vi "Worksheet to Dictionaries.vi"(8 "error in (no error)":errorcluster, 11 "Worksheet Data":T1) -> (0 "error out":errorcluster, 3 "Dictionaries Out":refnum<class "String Database.lvclass">[](array[class]))   [LabVIEW 2016, in "QPA TCF Parser.lvlib" / "QPA TCF Parser.lvclass"]
uses:
  QPA TCF Parser.lvclass
  Controls/Worksheet Data.ctl
  Plugins/String Database.lvlibp/String Database.lvclass
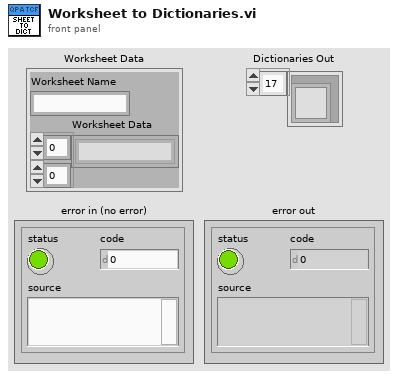
[diagram p1: front panel]
types:
  T1 = typedef "QPA TCF Parser.lvlib/QPA TCF Parser.lvclass/Worksheet Data.ctl" = cluster{"Worksheet Name":string, "Worksheet Data":string[][]}
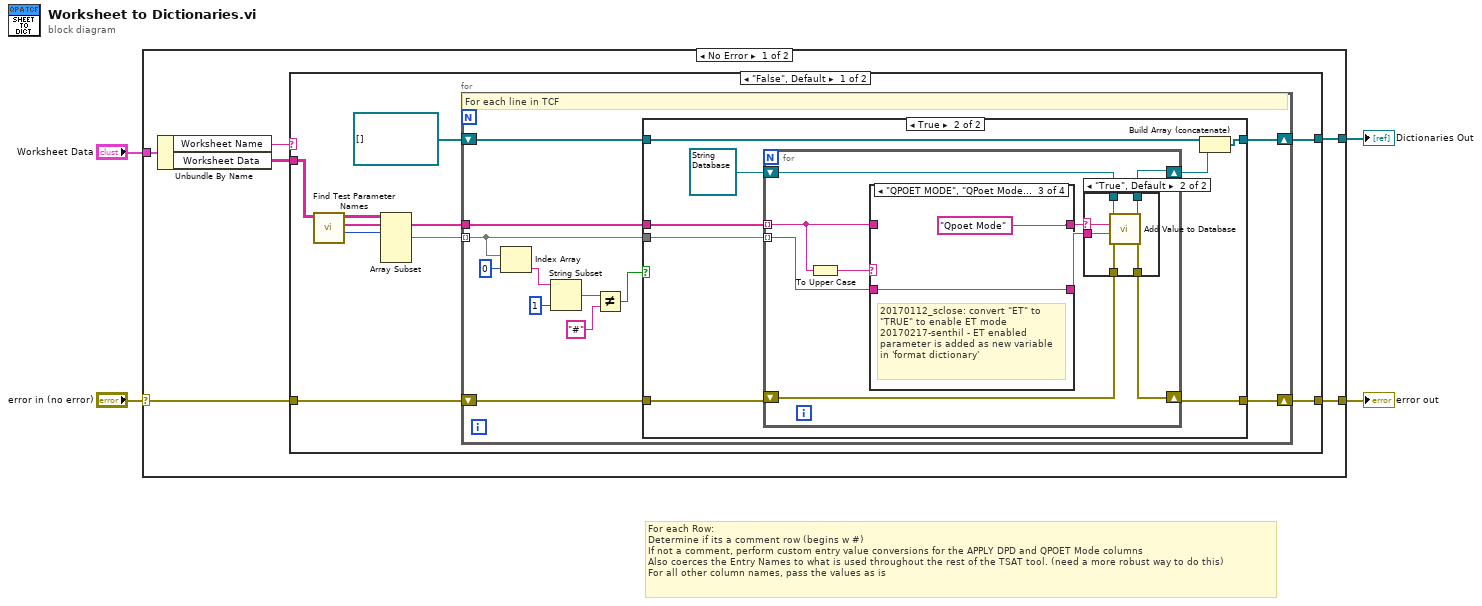
[diagram p0: block diagram]
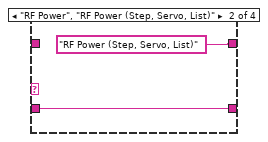
[diagram p4: hidden frame]
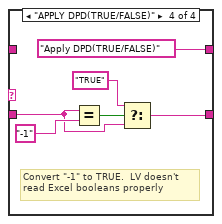
[diagram p5: hidden frame]
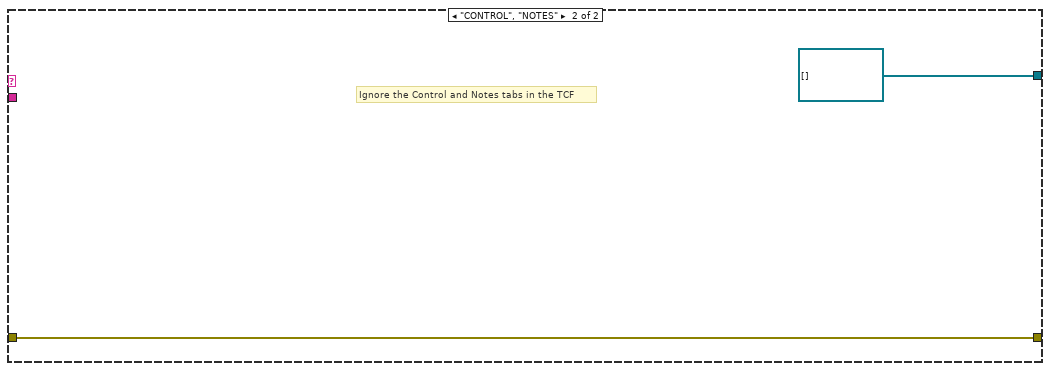
[diagram p7: hidden frame]
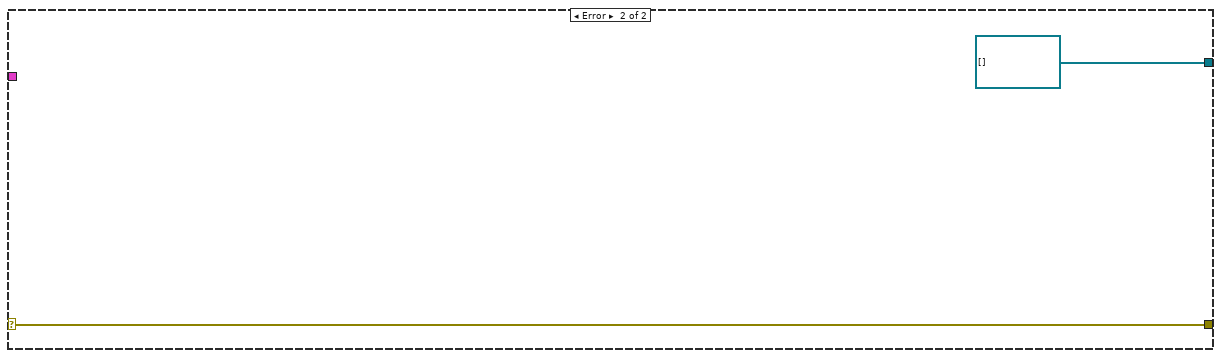
[diagram p8: hidden frame]
diagram:
  # "For each Row:\nDetermine if its a comment row (begins w #)\nIf not a comment, perform custom entry value conversions for the APPLY DPD and QPOET Mode columns\nAlso coerces the Entry Names to what is used throughout the rest of the TSAT tool. (need a more robust way to do this)\nFor all other column names, pass the values as is"
  n1 = case shown="No Error" "error in (no error)" {
    selector: "error in (no error)" -> [w9 w73]
    tunnel: [w10 w73] -> w4
    tunnel: "Worksheet Data" -> [w6 _]
    tunnel: [w5 refnum<class "String Database.lvclass">[] [] ("Dictionaries Out")] -> w1
    frame No Error {
      n2 = Unbundle By Name(w6) -> ("Worksheet Name"=w7:string, "Worksheet Data"=w8:string[][])
      n3 = case shown="\"False\", Default" w7 {
        tunnel: w8 -> [w19 _]
        tunnel: w9 -> [w14 w71]
        tunnel: [w13 w71] -> w10
        tunnel: [w11 refnum<class "String Database.lvclass">[] [] ("Dictionaries Out")] -> w5
        frame "False", Default {
          n4 = call "Find Test Parameter Names.vi"("Worksheet Data"=w19) -> ("Test Parameter Row Index"=w17:i32, "Test Parameters"=w15:string[], "Worksheet Data Out"=w18:string[][])  [unwired: 8 in]
          n5 = Array Subset(array=w18, index (row)=w17) -> (w16:string[][])  [unwired: 3 in]
          n6 = for {
            tunnel: w16 -> [w28] mode=indexing
            tunnel: w15 -> [w31]
            shift-right: [w29] -> w13
            shift-left: w14 -> [w30]
            shift-right: [w20] -> w11
            shift-left: refnum<class "String Database.lvclass">[] [] -> [w21]
            # "For each line in TCF"
            n7 = Index Array(array=w28, index=0) -> (element=w26:string)
            n8 = String Subset(string=w26, length (rest)=1 ("length (rest)")) -> (substring=w24:string)  [unwired: 1 in]
            n9 = Not Equal?(x=w24, y="#") -> (x != y?=w22:bool)
            n10 = case shown="True" w22 {
              tunnel: w31 -> [_ w41]
              tunnel: w30 -> [w33 w38]
              tunnel: [w33 w40] -> w29
              tunnel: w28 -> [_ w39]
              tunnel: w21 -> [w32 w35]
              tunnel: [w32 w34] -> w20
              frame False {
                # "Do Nothing on # comment"
              }
              frame True {
                n11 = for {
                  tunnel: w41 -> [w43] mode=indexing
                  tunnel: w39 -> [w46] mode=indexing
                  shift-right: [w48] -> w40
                  shift-left: w38 -> [w49]
                  shift-right: [w47] -> w36
                  shift-left: refnum<class "String Database.lvclass"> refnum ("String Database out") -> [w50]
                  n12 = To Upper Case(1:w43) -> (0:w44:string)
                  n13 = case shown="\"QPOET MODE\", \"QPoet Mode (Bypass, APT, EPT, ET)\"" w44 {
                    tunnel: w46 -> [w52 w54 w55 w59]
                    tunnel: [w52 w54 w55 w60] -> w45
                    tunnel: w43 -> [w51 _ _ _]
                    tunnel: [w51 "RF Power (Step, Servo, List)" ("Entry Name") "Qpoet Mode" ("Entry Name") "Apply DPD(TRUE/FALSE)" ("Entry Name")] -> w42
                    frame "", Default {
                    }
                    frame "RF Power", "RF Power (Step, Servo, List)" {
                    }
                    frame "QPOET MODE", "QPoet Mode (Bypass, APT, EPT, ET)" {
                      # "20170112_sclose: convert \"ET\" to \n\"TRUE\" to enable ET mode\n20170217-senthil - ET enabled \nparameter is added as new variable\nin 'format dictionary'"
                    }
                    frame "APPLY DPD(TRUE/FALSE)" {
                      # "Convert \"-1\" to TRUE.  LV doesn't\nread Excel booleans properly"
                      n14 = Equal?(x=w59, y="-1") -> (x = y?=w61:bool)
                      n15 = Select(t="TRUE", s=w61, f=w59) -> (s? t:f=w60:string)
                    }
                  }
                  n16 = case shown="\"True\", Default" w42 {
                    selector: w42 -> [_ w67]
                    tunnel: w50 -> [w64 w70]
                    tunnel: w49 -> [w63 w69]
                    tunnel: [w63 w68] -> w48
                    tunnel: w45 -> [_ w66]
                    tunnel: [w64 w65] -> w47
                    frame "" {
                    }
                    frame "True", Default {
                      n17 = call "Add Value to Database.vi"("error in (no error)"=w69, "Entry Value"=w66, "Entry Name"=w67, "Dictionary In"=w70) -> ("error out"=w68:errorcluster, "Dictionary Out"=w65:refnum<class "String Database.lvclass">)  [unwired: 5 in, 1 out]
                    }
                  }
                }
                n18 = Build Array (concatenate)(w35, w36) -> (w34:refnum<class "String Database.lvclass">[])
              }
            }
          }
        }
        frame "CONTROL", "NOTES" {
          # "Ignore the Control and Notes tabs in the TCF"
        }
      }
    }
    frame Error {
    }
  }
  "error out" <- w4
  "Dictionaries Out" <- w1
